vi "get log configure.vi"(8 "error in (no error)":errorcluster) -> (0 "error out":errorcluster, 2 "log options":T1, 3 "default":bool)   [LabVIEW 2024, in "atsj peakcan basic.lvlib"]
uses:
  atsj peakcan basic.lvlib
  log options.ctl
  parameter.ctl
  get parameter - i32.vi
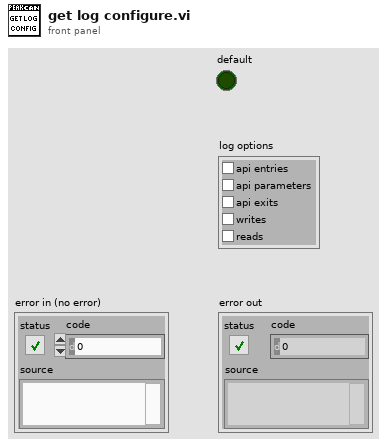
[diagram p1: front panel]
types:
  T1 = typedef "atsj peakcan basic.lvlib/log options.ctl" = cluster{"api entries":bool, "api parameters":bool, "api exits":bool, "writes":bool, "reads":bool}
  T2 = typedef "atsj peakcan basic.lvlib/parameter.ctl" = enum8{"DEVICE_ID", "5VOLTS_POWER", "RECEIVE_EVENT", "MESSAGE_FILTER", "API_VERSION", "CHANNEL_VERSION", "BUSOFF_AUTORESET", "LISTEN_ONLY", "LOG_LOCATION", "LOG_STATUS", "LOG_CONFIGURE", "LOG_TEXT", "CHANNEL_CONDITION", "HARDWARE_NAME", "RECEIVE_STATUS", "CONTROLLER_NUMBER", "TRACE_LOCATION", "TRACE_STATUS", "TRACE_SIZE", "TRACE_CONFIGURE", "CHANNEL_IDENTIFYING", "CHANNEL_FEATURES", "BITRATE_ADAPTING", "BITRATE_INFO", "BITRATE_INFO_FD", "BUSSPEED_NOMINAL", "BUSSPEED_DATA", "IP_ADDRESS", "LAN_SERVICE_STATUS", "ALLOW_STATUS_FRAMES", "ALLOW_RTR_FRAMES", "ALLOW_ERROR_FRAMES", "INTERFRAME_DELAY", "ACCEPTANCE_FILTER_11BIT", "ACCEPTANCE_FILTER_29BIT", "IO_DIGITAL_CONFIGURATION", "IO_DIGITAL_VALUE", "IO_DIGITAL_SET", "IO_DIGITAL_CLEAR", "IO_ANALOG_VALUE", "FIRMWARE_VERSION", "ATTACHED_CHANNELS_COUNT", "ATTACHED_CHANNELS", "ALLOW_ECHO_FRAMES", "DEVICE_PART_NUMBER", "HARD_RESET_STATUS", "LAN_CHANNEL_DIRECTION", "DEVICE_GUID"}
  T3 = cluster{"Boolean array[0]":bool, "Boolean array[1]":bool, "Boolean array[2]":bool, "Boolean array[3]":bool, "Boolean array[4]":bool}
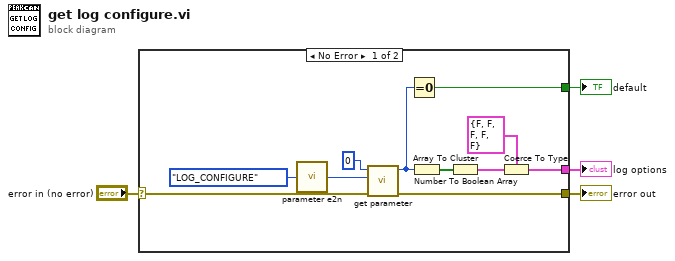
[diagram p0: block diagram]
diagram:
  n1 = case shown="No Error" "error in (no error)" {
    selector: "error in (no error)" -> [w12 w16]
    tunnel: [w11 w16] -> w3
    tunnel: [w8 _] -> w2
    tunnel: [w5 _] -> w1
    frame No Error {
      n2 = call "parameter e2n.vi"("parameter"=parameter."LOG_CONFIGURE") -> ("number"=w13:u8)
      n3 = call-poly "get parameter.vi"("error in (no error)"=w12, "parameter"=w13, "channel"=u16 0) -> ("error out"=w11:errorcluster, "value"=w6:i32)  [unwired: 7 in]
      n4 = Equal To 0?(x=w6) -> (x = 0?=w5:bool)
      n5 = Number To Boolean Array(number=w6) -> (Boolean array=w10:bool[])
      n6 = Array To Cluster(array=w10) -> (cluster=w9:T3)
      n7 = Coerce To Type(0:w9, 1:T1 {"api entries"=FALSE, "api parameters"=FALSE, "api exits"=FALSE, "writes"=FALSE, "reads"=FALSE}) -> (2:w8:T1)
    }
    frame Error {
    }
  }
  "error out" <- w3
  "default" <- w1
  "log options" <- w2
